vi "write system hardware ref.vi"(8 "error in":errorcluster, 10 "system hardware ref":refnum<data-value>, 11 "controller in":refnum<class "Controller.lvclass">) -> (0 "error out":errorcluster, 3 "controller out":refnum<class "Controller.lvclass">)   [LabVIEW 2014, in "SMI.lvlib" / "Controller.lvclass"]
uses:
  Controller.lvclass
  Controller.lvclass/Controller.ctl
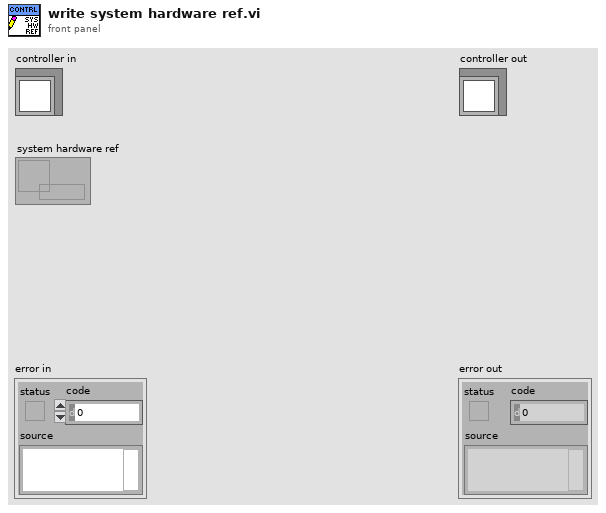
[diagram p1: front panel]
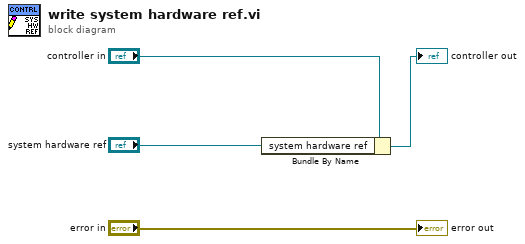
[diagram p0: block diagram]
diagram:
  n1 = Bundle By Name(cluster="controller in", "system hardware ref"="system hardware ref") -> (→"controller out":refnum<class "Controller.lvclass">)
  "error out" <- "error in"
